vi "Delete Background.vi"(8 "error in":errorcluster, 11 "Image Pixels (Float) in":sgl[][](array[numeric])) -> (0 "error out":errorcluster, 3 "Image Pixels (Float) out":sgl[][](array[numeric]))   [LabVIEW 2018]
uses:
  <userlib>/_OpenG.lib/array/array.llb/Delete Elements from 2D Array (SGL)__ogtk.vi
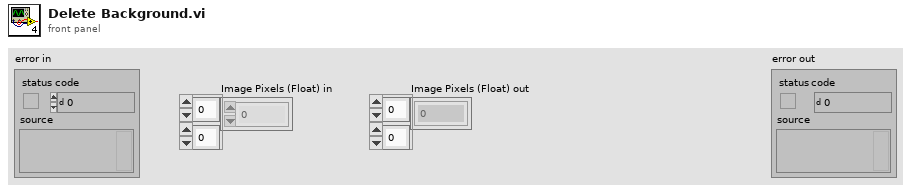
[diagram p1: front panel]
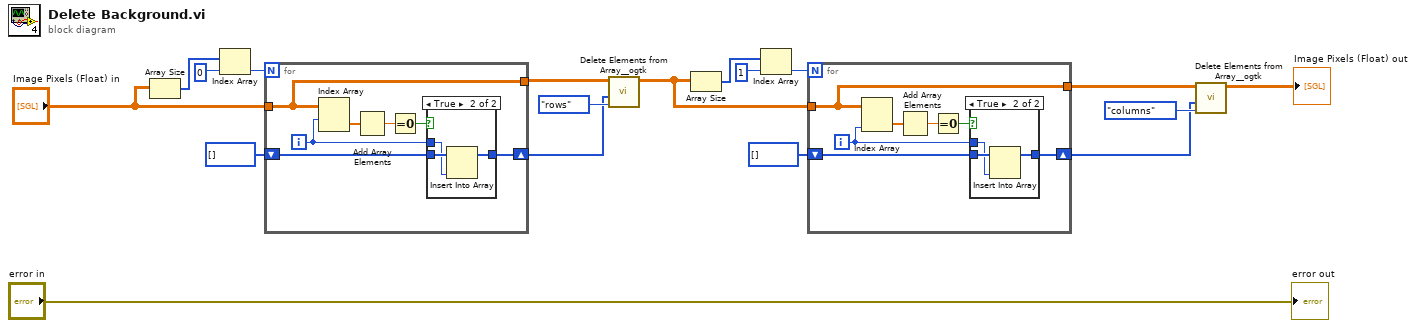
[diagram p0: block diagram]
diagram:
  n1 = Array Size(array="Image Pixels (Float) in") -> (size(s)=w15:i32[])
  n2 = Index Array(array=w15, index=0) -> (element=w12:i32)
  n3 = for {
    N: w12 -> [_]
    shift-right: [w22] -> w9
    shift-left: i32[] [] -> [w23]
    tunnel: "Image Pixels (Float) in" -> [w19]
    tunnel: [w19] -> w11
    i -> [w20]
    n4 = Index Array(array=w19, index (row)=w20) -> (element=w25:sgl[])  [unwired: 1 in]
    n5 = Add Array Elements(numeric array=w25) -> (sum=w24:sgl)
    n6 = Equal To 0?(x=w24) -> (x = 0?=w21:bool)
    n7 = case shown="True" w21 {
      tunnel: w23 -> [w26 w29]
      tunnel: [w26 w28] -> w22
      tunnel: w20 -> [_ w27]
      frame False {
      }
      frame True {
        n8 = Insert Into Array(array=w29, new element=w27) -> (w28:i32[])  [unwired: 1 in]
      }
    }
  }
  n9 = call-poly <userlib>:"Delete Elements from Array__ogtk.vi"("delete (rows or columns)"=enum16{"rows", "columns"}."rows", "indices"=w9, "array"=w11) -> ("array w/ subset deleted"=w7:sgl[][])  [unwired: 7 in, 1 out]
  n10 = Array Size(array=w7) -> (size(s)=w17:i32[])
  n11 = Index Array(array=w17, index=1) -> (element=w8:i32)
  n12 = for {
    N: w8 -> [_]
    shift-right: [w34] -> w3
    shift-left: i32[] [] -> [w35]
    tunnel: w7 -> [w31]
    tunnel: [w31] -> w4
    i -> [w32]
    n13 = Index Array(array=w31, index (col)=w32) -> (element=w30:sgl[])  [unwired: 1 in]
    n14 = Add Array Elements(numeric array=w30) -> (sum=w36:sgl)
    n15 = Equal To 0?(x=w36) -> (x = 0?=w33:bool)
    n16 = case shown="True" w33 {
      tunnel: w35 -> [w37 w40]
      tunnel: [w37 w39] -> w34
      tunnel: w32 -> [_ w38]
      frame False {
      }
      frame True {
        n17 = Insert Into Array(array=w40, new element=w38) -> (w39:i32[])  [unwired: 1 in]
      }
    }
  }
  n18 = call-poly <userlib>:"Delete Elements from Array__ogtk.vi"("delete (rows or columns)"=enum16{"rows", "columns"}."columns", "indices"=w3, "array"=w4) -> ("array w/ subset deleted"=→"Image Pixels (Float) out":sgl[][])  [unwired: 7 in, 1 out]
  "error out" <- "error in"
